vi "Configure DMRS For Mapping Type B.vi"(4 "Max Length (1)":i32=1, 5 "Additional Position (0)":i32, 6 "Config Type (1)":i32=1, 7 "Bandwidth Part (BWP0)":T2 items=["BWP0"], 8 "error in (no error)":errorcluster, 9 "Carrier Component (1)":T1=1, 10 "Instance (1)":T3=1, 11 "VISA resource name":refnum<visa-resource-name>) -> (0 "error out":errorcluster, 3 "VISA resource name out":refnum<visa-resource-name>)   [LabVIEW 2020, in "Rohde&Schwarz CMXP NR FR2 Measurement.lvlib"]
doc: "Configures the DM-RS for mapping type B.\n\nAttribute:\nRSCMXPNRFR2M_ATTR_DMRS_FOR_MAPPING_TYPE_B\n\nRemote-control command:\nCONFigure:NRMMw:MEAS<i>[:CC<no>]:BWPart:PUSCh:DMTB"
uses:
  <instrlib>/Rohde&Schwarz CMXP NR FR2 Measurement/Rohde&Schwarz CMXP NR FR2 Measurement.lvlib
  <instrlib>/Rohde&Schwarz CMXP NR FR2 Measurement/Private/_Instance.ctl
  <instrlib>/Rohde&Schwarz CMXP NR FR2 Measurement/Private/_Bandwidth Part.ctl
  <instrlib>/Rohde&Schwarz CMXP NR FR2 Measurement/Private/_Carrier Component.ctl
  <instrlib>/Rohde&Schwarz CMXP NR FR2 Measurement/Private/rsidr_core.llb/rsidr_core.lvlib
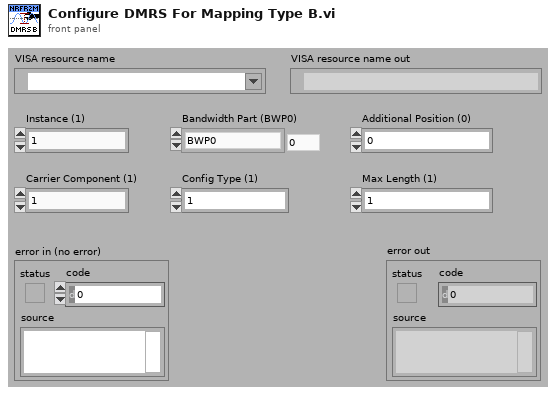
[diagram p1: front panel]
types:
  T1 = typedef "Rohde&Schwarz CMXP NR FR2 Measurement.lvlib/_Carrier Component.ctl" = i32
  T2 = typedef "Rohde&Schwarz CMXP NR FR2 Measurement.lvlib/_Bandwidth Part.ctl" = i32
  T3 = typedef "Rohde&Schwarz CMXP NR FR2 Measurement.lvlib/_Instance.ctl" = i32
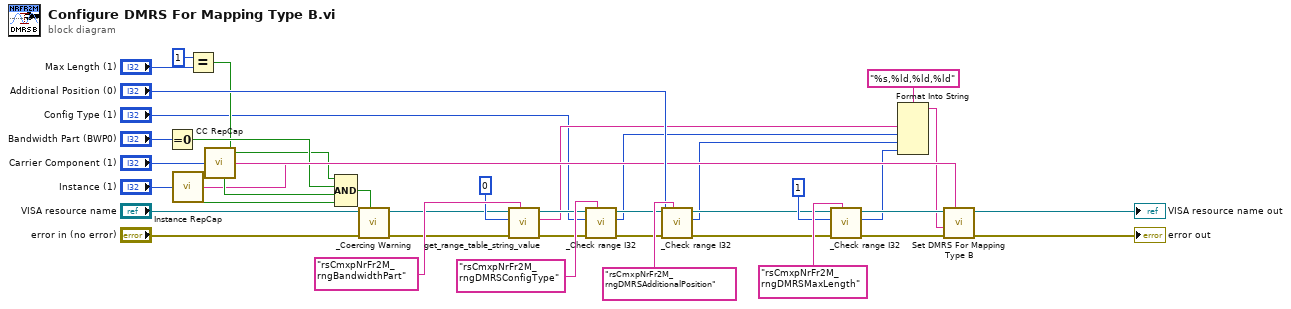
[diagram p0: block diagram]
diagram:
  n1 = Equal To 0?(x="Bandwidth Part (BWP0)") -> (x = 0?=w6:bool)
  n2 = call <instrlib>:"Instance RepCap.vi"("Instance In"="Instance (1)") -> ("In Range?"=w32:bool, "RepCap Identifier Out"=w3:string)  [unwired: 1 in]
  n3 = Equal?(x=1, y="Max Length (1)") -> (x = y?=w5:bool)
  n4 = call <instrlib>:"CC RepCap.vi"("CC In"="Carrier Component (1)", "RepCap String In (\"\")"=w3) -> ("In Range?"=w31:bool, "RepCap Identifier Out"=w15:string)
  n5 = Compound Arithmetic op=AND(w5, w6, w31, w32) -> (w34:bool)
  n6 = call <instrlib>:"_Coercing Warning.vi"("In Range?"=w34, "error in (no error)"="error in (no error)", "VISA resource name"="VISA resource name") -> ("error out"=w28:errorcluster, "VISA resource name out"=w29:refnum<visa-resource-name>)  [unwired: 7 in]
  n7 = call <instrlib>:"get_range_table_string_value.vi"("Range Table ID in"="rsCmxpNrFr2M_rngBandwidthPart", "error in"=w28, "I32 input"=0, "VISA resource name"=w29) -> ("error out"=w17:errorcluster, "String Value out"=w10:string, "VISA resource name out"=w16:refnum<visa-resource-name>)  [unwired: 5 in]
  n8 = call <instrlib>:"_Check range I32.vi"("Range Table Identifier"="rsCmxpNrFr2M_rngDMRSConfigType", "error in (no error)"=w17, "I32 Value In"="Config Type (1)", "VISA resource name"=w16) -> ("error out"=w24:errorcluster, "I32 Value Out"=w9:i32, "VISA resource name out"=w23:refnum<visa-resource-name>)  [unwired: 5 in]
  n9 = call <instrlib>:"_Check range I32.vi"("Range Table Identifier"="rsCmxpNrFr2M_rngDMRSAdditionalPosition", "error in (no error)"=w24, "I32 Value In"="Additional Position (0)", "VISA resource name"=w23) -> ("error out"=w20:errorcluster, "I32 Value Out"=w8:i32, "VISA resource name out"=w19:refnum<visa-resource-name>)  [unwired: 5 in]
  n10 = call <instrlib>:"_Check range I32.vi"("Range Table Identifier"="rsCmxpNrFr2M_rngDMRSMaxLength", "error in (no error)"=w20, "I32 Value In"=1, "VISA resource name"=w19) -> ("error out"=w14:errorcluster, "I32 Value Out"=w7:i32, "VISA resource name out"=w13:refnum<visa-resource-name>)  [unwired: 5 in]
  n11 = Format Into String(format string="%s,%ld,%ld,%ld", w10, w9, w8, w7) -> (resulting string=w2:string)  [unwired: 2 in, 1 out]
  n12 = call "Set DMRS For Mapping Type B"("Repeated Capabilities"=w15, "error in (no error)"=w14, "DMRS For Mapping Type B ()"=w2, "instrument handle"=w13) -> ("error out"=→"error out":errorcluster, "instrument handle out"=→"VISA resource name out":refnum<visa-resource-name>)  [unwired: 6 in]
